vi "UART Send.vi"(0 "UART Ref In":T1={"FPGA I/O"="Mod1/DIO0", "Buffer Ref"="", "Stop Ref"=""}, 7 "Baud Rate (9600)":u32=9600) -> ()   [LabVIEW 2016, in "UART 8N1 (FPGA).lvlib"]
uses:
  UART 8N1 (FPGA).lvlib
  UART Ref.ctl
  TxD CMD.ctl
  <vilib>/Platform/TimedLoop/XDataNode/timing_clust.ctl
  <vilib>/Platform/TimedLoop/XDataNode/nitl_modes.ctl
  <vilib>/Platform/TimedLoop/XDataNode/wakeup.ctl
  <vilib>/rvi/Emulation/niFpgaSctlEmulationGetInTimedLoop.vi
  <vilib>/rvi/Emulation/niFpgaEmulationReportErrorSimple.vi
  <vilib>/rvi/Emulation/niFpgaGetClockAttributes.vi
  <vilib>/rvi/Emulation/niFpgaCriticalErrorInLSC.vi
  <vilib>/rvi/eio/common/nirviEmuTemplateMethod_errors.vi
  <vilib>/rvi/DataTransferAndStorage/Container/Common/niFpgaContainerExecOnDevCompGetState.vi
  <vilib>/rvi/Emulation/niFpgaEmulationIsFPGAContextNoSignature.vi
  <vilib>/rvi/DataTransferAndStorage/Container/Common/niFpgaContainerGetUniqueNameForEmu.vi
  <vilib>/rvi/Memory/Memory_Emulation/niFpgaMemoryEmulationCacheClearOnFirstRun.vi
  <vilib>/rvi/Memory/Memory_Emulation/nirvimemoryEmulationManagerCache_MakeExclusive.vi
  <vilib>/rvi/Memory/Memory_Emulation/niFpgaMemoryEmulationValidateCache.vi
  <vilib>/rvi/Memory/Memory_Emulation/nirvimemoryEmulationManagerCache_InsertValue.vi
  <vilib>/Utility/error.llb/Clear Errors.vi
  <vilib>/rvi/Memory/Memory_Emulation/nirvimemoryEmulationManagerCache_ReleaseExclusive.vi
  <vilib>/rvi/Memory/Memory_Emulation/nirvimemoryEmulationManagerCache_GetValue.vi
  <vilib>/rvi/Memory/Memory_Emulation/nirvimemoryEmulationManagerCache_SetValue.vi
  <vilib>/rvi/Emulation/niFpgaProcessEmulError.vi
  <vilib>/rvi/errors/niFpgaSetErrorForExecOnDevCompSimple.vi
  <vilib>/rvi/eio/common/nirviEmuReportErrorAndStop.vi
  <vilib>/rvi/FIFO/Fifo_Resource/nirvififoEmulationSetSize.vi
  <vilib>/rvi/FIFO/Fifo_Resource/nirviFifoEmulationQueueMgr.vi
  <instcachedir>/0/nirviFifoEmulationQueueMgr_E5CAEC123FF24DC58D834DCA3CDAA9B5.lvgen/nirviFifoEmulationQueueMgr_E5CAEC123FF24DC58D834DCA3CDAA9B5_000.vi
  <vilib>/rvi/FIFO/Fifo_Resource/nirvififoEmulationDetermineInputValidOut.vi
  <vilib>/rvi/FIFO/Fifo_Resource/nirvififoEmulationCreateLock.vi
  <vilib>/rvi/FIFO/Fifo_Resource/nirvififoEmulationObtainLock.vi
  <vilib>/rvi/FIFO/Fifo_Resource/nirvififoEmulationReleaseLock.vi
  <vilib>/rvi/occurrence/nirviWaitOnOccurrenceBase.vi
  <vilib>/rvi/errors/nirviReportUnexpectedCaseInternalError.vi
  <vilib>/rvi/errors/nirviReportUnexpectedCaseInternalError (U32).vi
  <vilib>/rvi/interface/RandomDataEmulation/niFpgaRandomDataHandleErrors.vi
  <vilib>/Platform/TimedLoop/XDataNode/XDataNode.xnode
  <vilib>/eio/EIONode/EIONode.xnode
  <vilib>/rvi/DataTransferAndStorage/Container/XNode/niFpgaContainer.xnode
  <vilib>/rvi/DataTransferAndStorage/Register/Emulation/niFpgaRegisterEmulationRefIn.vi
  <vilib>/rvi/FIFO/Fifo_Resource/niFpgaFifoEmulationRefIn.vi
  <vilib>/Platform/TimedLoop/XDataNode/XDNodeRunTimeDep.lvlib
panel:
  # "UART Send\nTxD, 8N1"
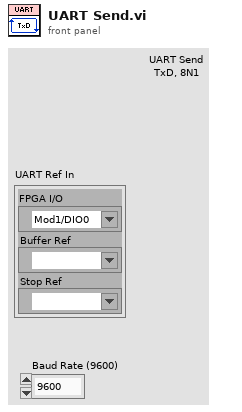
[diagram p1: front panel]
types:
  T1 = typedef "UART 8N1 (FPGA).lvlib/UART Ref.ctl" = cluster{"FPGA I/O":refnum<k21>, "Buffer Ref":refnum<k21>, "Stop Ref":refnum<k21>}
  T2 = typedef "UART 8N1 (FPGA).lvlib/TxD CMD.ctl" = enum16{"Init", "Idle", "Write Start Bit", "Wait One Bit (Start)", "Write Data Bit", "Wait One Bit (Data)", "Write Stop Bit", "Wait One Bit (Stop)", "Close"}
  T3 = typedef "XDNodeRunTimeDep.lvlib/timing_clust.ctl" = cluster{"Expected End [f-1]":u64, "Actual End [f-1]":u64, "Finished Late? [f-1]":bool, "Expected End [i-1]":u64, "Actual End [i-1]":u64, "Finished Late? [i-1]":bool, "Expected Start [i]":u64, "Actual Start [i]":u64, "Expected Start [f]":u64, "Actual Start [f]":u64, "Source Name":string, "Structure Name":string, "Period":i64, "Deadline":i64, "Offset":i64, "Start":i64, "Priority":i32, "Timeout":i32, "Mode":T4, "Wakeup Reason":T5, "Error":errorcluster, "Source Type":string, "Secondary Source Type":string, "Global End Time":u64, "Global Start Time":u64, "Frame Duration":u64, "Iteration Duration":u64, "Assigned CPU":i32, "I/O Scan Engine Mode":u32}
  T4 = typedef "XDNodeRunTimeDep.lvlib/nitl_modes.ctl" = enum32{"No Change", "Process missed periods, maintain original phase", "Discard missed periods, maintain original phase", "Process missed periods, ignore original phase", "Discard missed periods, ignore original phase"}
  T5 = typedef "XDNodeRunTimeDep.lvlib/wakeup.ctl" = enum32{"Normal", "Aborted", "Asynchronous wakeup", "Timing source error", "Timed loop error", "Timeout"}
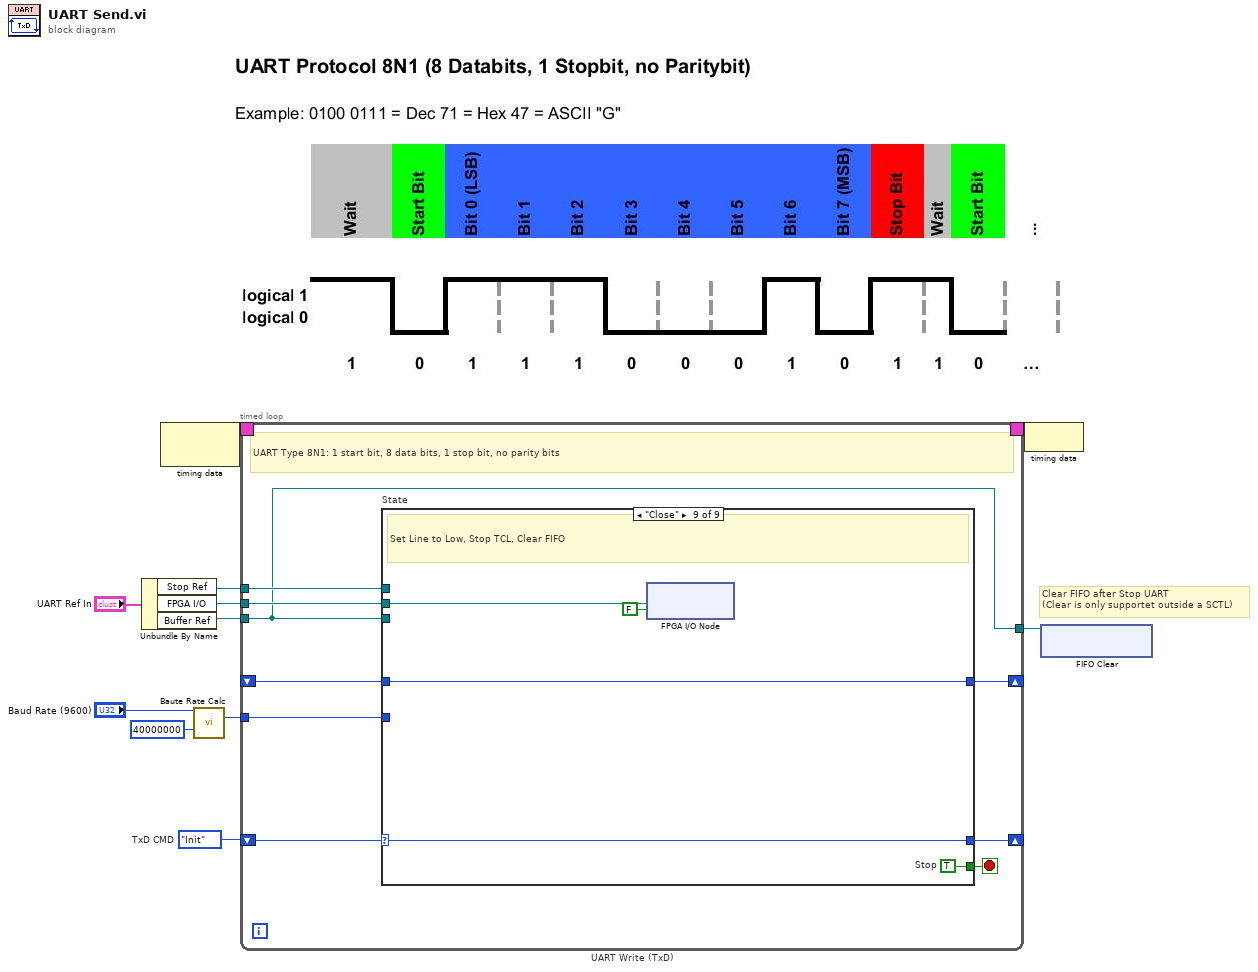
[diagram p0: block diagram]
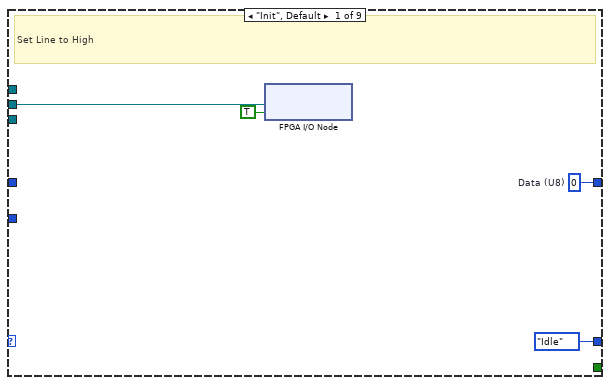
[diagram p2: hidden frame]
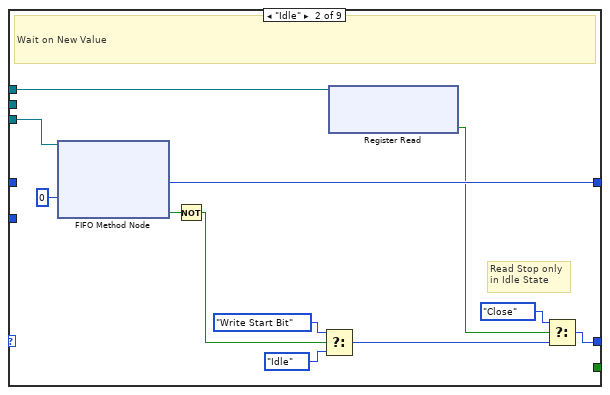
[diagram p3: hidden frame]
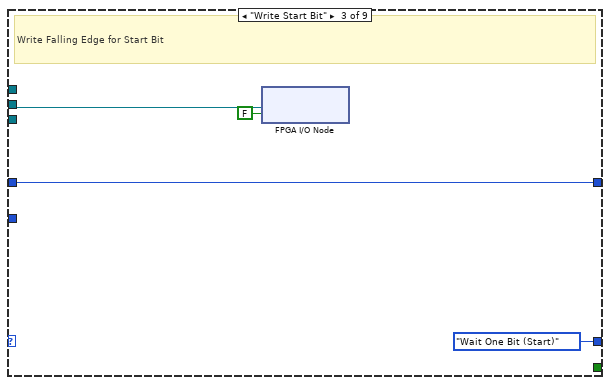
[diagram p4: hidden frame]
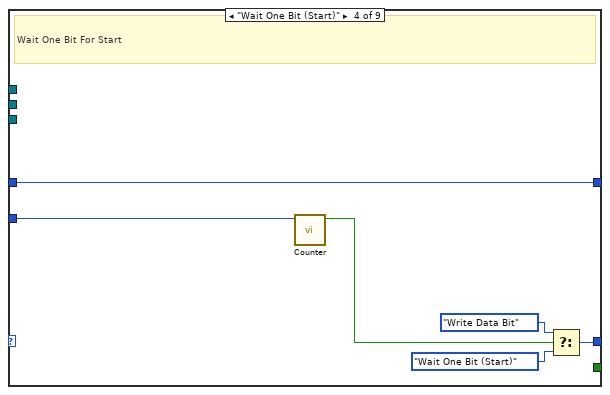
[diagram p5: hidden frame]
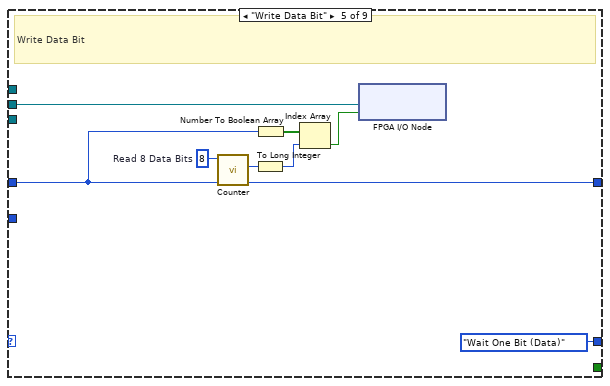
[diagram p6: hidden frame]
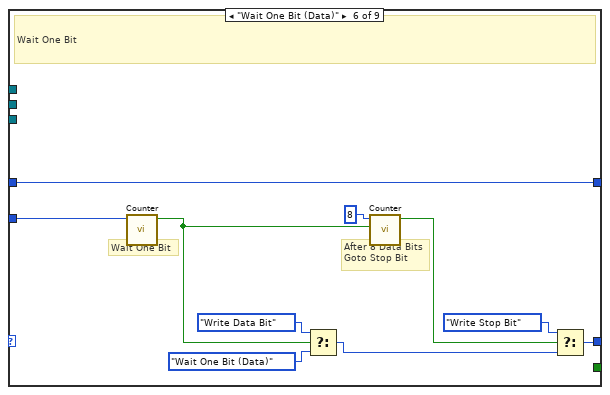
[diagram p7: hidden frame]
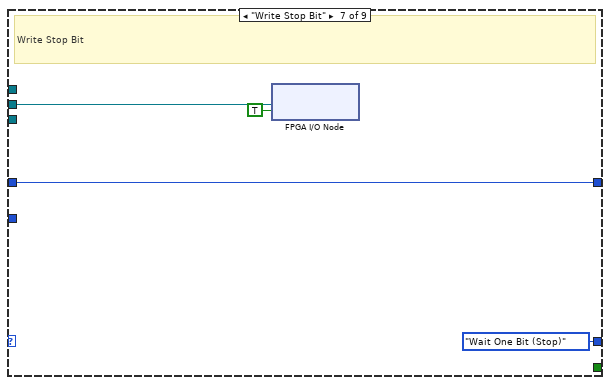
[diagram p8: hidden frame]
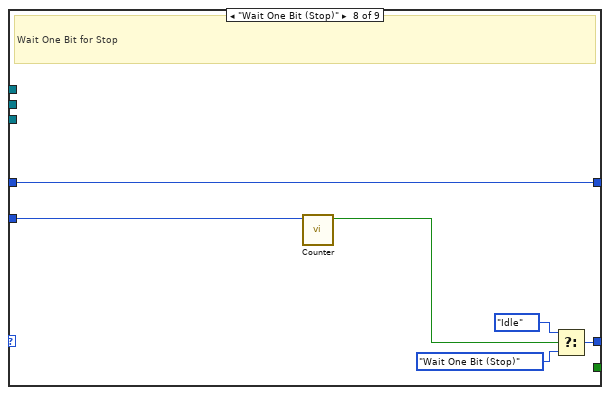
[diagram p9: hidden frame]
diagram:
  w9 = TxD_CMD."Init"  # TxD CMD
  # "Clear FIFO after Stop UART\n(Clear is only supportet outside a SCTL)"
  n1 = Unbundle By Name("UART Ref In") -> ("Stop Ref"=w5:refnum<k21>, "FPGA I/O"=w8:refnum<k21>, "Buffer Ref"=w7:refnum<k21>)
  n2 = node-c288() -> (w11:T3)  [unwired: 1 in]
  n3 = call "Baute Rate Calc.vi"("Baud Rate (9600)"="Baud Rate (9600)", "FPGA Clock Rate (40000000)"=u32 40000000) -> ("One Bit"=w1:u32)  [unwired: 10 in, 3 out]
  n4 = timed-loop "UART Write (TxD)" {
    timing: w11 -> [_]
    timing-out: [_] -> w10
    shift-right: [w16] -> _
    shift-left: w9 -> [w14]
    tunnel: w8 -> [w20]
    shift-right: [w18] -> _
    shift-left: _ -> [w17]
    tunnel: w1 -> [w15]
    tunnel: w7 -> [w12]
    tunnel: w5 -> [w13]
    tunnel: [w12] -> w4
    stop <- w19 stop-if-true
    # "UART Type 8N1: 1 start bit, 8 data bits, 1 stop bit, no parity bits"
    n5 = case "State" shown="\"Close\"" w14 {
      selector: w14 -> [_ _ _ _ _ _ _ _ w77]
      tunnel: w20 -> [w22 _ w38 _ w54 _ w65 _ w75]
      tunnel: [_ _ _ _ _ _ _ _ w79] -> w19
      tunnel: [TxD_CMD."Idle" ("TxD State") w28 TxD_CMD."Wait One Bit (Start)" ("TxD State") w43 TxD_CMD."Wait One Bit (Data)" ("TxD State") w56 TxD_CMD."Wait One Bit (Stop)" ("TxD State") w70 w77] -> w16
      tunnel: [w23 w31 w40 w44 w52 w64 w68 w74 w78] -> w18
      tunnel: w17 -> [_ _ w40 w44 w52 w64 w68 w74 w78]
      tunnel: w15 -> [_ _ _ w41 _ w55 _ w69 _]
      tunnel: w12 -> [_ w30 _ _ _ _ _ _ _]
      tunnel: w13 -> [_ w26 _ _ _ _ _ _ _]
      frame "Init", Default {
        w23 = u8 0  # Data (U8)
        # "Set Line to High"
        n6 = xnode "FPGA I/O Node"("I/O Item"=TRUE, "FPGA I/O In"=w22) -> ()  [unwired: 1 out]
      }
      frame "Idle" {
        # "Read Stop only\nin Idle State"
        # "Wait on New Value"
        n7 = xnode ("FIFO Method Node")("Timeout"=0, "FIFO In"=w30) -> ("Element"=w31:u8, "Timed Out?"=w33:bool)  [unwired: 1 out]
        n8 = Not(x=w33) -> (.not. x?=w32:bool)
        n9 = Select(t=TxD_CMD."Write Start Bit", s=w32, f=TxD_CMD."Idle" ("TxD State")) -> (s? t:f=w27:T2)
        n10 = xnode ("Register Read")("Register In"=w26) -> ("Data"=w25:bool)  [unwired: 1 out]
        n11 = Select(t=TxD_CMD."Close", s=w25, f=w27) -> (s? t:f=w28:T2)
      }
      frame "Write Start Bit" {
        # "Write Falling Edge for Start Bit"
        n12 = xnode "FPGA I/O Node"("I/O Item"=FALSE, "FPGA I/O In"=w38) -> ()  [unwired: 1 out]
      }
      frame "Wait One Bit (Start)" {
        # "Wait One Bit For Start"
        n13 = call "Counter.vi"("Counter End  Value"=w41) -> ("End Reached"=w42:bool)  [unwired: 9 in, 1 out]
        n14 = Select(t=TxD_CMD."Write Data Bit", s=w42, f=TxD_CMD."Wait One Bit (Start)" ("TxD State")) -> (s? t:f=w43:T2)
      }
      frame "Write Data Bit" {
        w53 = u32 8  # Read 8 Data Bits
        # "Write Data Bit"
        n15 = call "Counter.vi"("Counter End  Value"=w53) -> ("Counter Value"=w49:u32)  [unwired: 9 in, 1 out]
        n16 = To Long Integer(number=w49) -> (32bit integer=w48:i32)
        n17 = Number To Boolean Array(number=w52) -> (Boolean array=w51:bool[])
        n18 = Index Array(array=w51, index=w48) -> (element=w50:bool)
        n19 = xnode "FPGA I/O Node"("I/O Item"=w50, "FPGA I/O In"=w54) -> ()  [unwired: 1 out]
      }
      frame "Wait One Bit (Data)" {
        # "After 8 Data Bits\nGoto Stop Bit"
        # "Wait One Bit"
        # "Wait One Bit"
        n20 = call "Counter.vi"("Counter End  Value"=w55) -> ("End Reached"=w61:bool)  [unwired: 9 in, 1 out]
        n21 = Select(t=TxD_CMD."Write Data Bit", s=w61, f=TxD_CMD."Wait One Bit (Data)" ("TxD State")) -> (s? t:f=w58:T2)
        n22 = call "Counter.vi"("Input Valid"=w61, "Counter End  Value"=u32 8) -> ("End Reached"=w57:bool)  [unwired: 8 in, 1 out]
        n23 = Select(t=TxD_CMD."Write Stop Bit", s=w57, f=w58) -> (s? t:f=w56:T2)
      }
      frame "Write Stop Bit" {
        # "Write Stop Bit"
        n24 = xnode "FPGA I/O Node"("I/O Item"=TRUE, "FPGA I/O In"=w65) -> ()  [unwired: 1 out]
      }
      frame "Wait One Bit (Stop)" {
        # "Wait One Bit for Stop"
        n25 = call "Counter.vi"("Counter End  Value"=w69) -> ("End Reached"=w73:bool)  [unwired: 9 in, 1 out]
        n26 = Select(t=TxD_CMD."Idle", s=w73, f=TxD_CMD."Wait One Bit (Stop)" ("TxD State")) -> (s? t:f=w70:T2)
      }
      frame "Close" {
        w79 = TRUE  # Stop
        # "Set Line to Low, Stop TCL, Clear FIFO"
        n27 = xnode "FPGA I/O Node"("I/O Item"=FALSE, "FPGA I/O In"=w75) -> ()  [unwired: 1 out]
      }
    }
  }
  n28 = node-c288(w10) -> ()
  n29 = xnode ("FIFO Clear")("FIFO In"=w4) -> ()  [unwired: 1 out]
